vi "Read Valid Pixels Top Left.vi"(8 "error in (no error)":errorcluster, 11 "ImageRectifier in":refnum<class "ImageRectifier.lvclass">) -> (0 "error out":errorcluster, 2 "Image Point":T1, 3 "ImageRectifier out":refnum<class "ImageRectifier.lvclass">)   [LabVIEW 2020, in "image.lvlib" / "ImageRectifier.lvclass"]
uses:
  ImageRectifier.lvclass
  common/Image Point (Integer).ctl
  ImageRectifier.lvclass/ImageRectifier.ctl
  common/common.lvlib
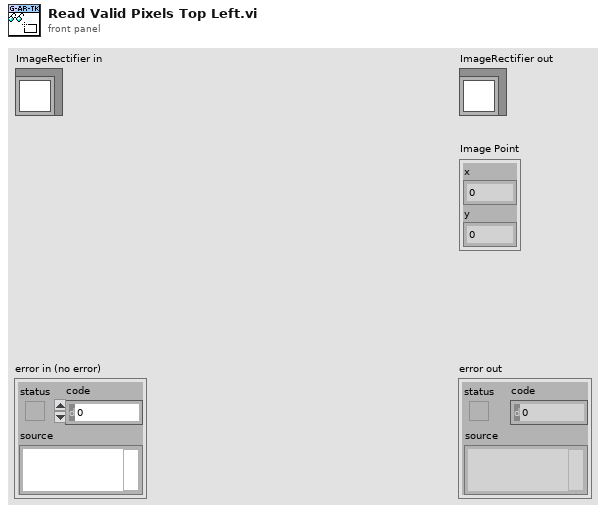
[diagram p1: front panel]
types:
  T1 = typedef "common.lvlib/Image Point (Integer).ctl" = cluster{"x":i32, "y":i32}
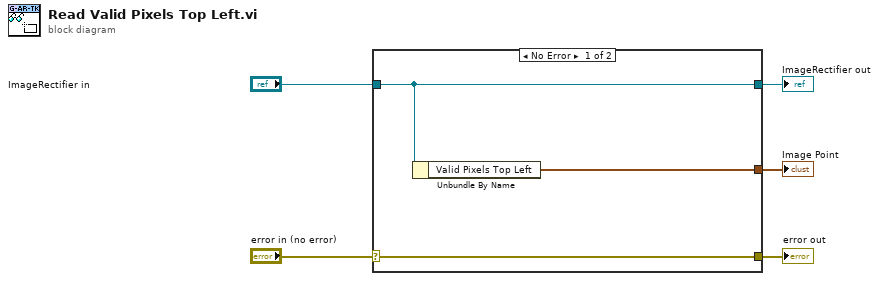
[diagram p0: block diagram]
diagram:
  n1 = case shown="No Error" "error in (no error)" {
    selector: "error in (no error)" -> [w8 w9]
    tunnel: [w8 w9] -> w4
    tunnel: [w7 w10] -> w2
    tunnel: "ImageRectifier in" -> [w7 w10]
    tunnel: [w6 _] -> w1
    frame No Error {
      n2 = Unbundle By Name(w7) -> ("Valid Pixels Top Left"=w6:T1)
    }
    frame Error {
    }
  }
  "error out" <- w4
  "ImageRectifier out" <- w2
  "Image Point" <- w1
